vi "free tls config.vi"(8 "error in":errorcluster, 11 "config":u64) -> (0 "error out":errorcluster)   [LabVIEW 2016, in "lv tls dll.lvlib"]
uses:
  lv tls dll.lvlib
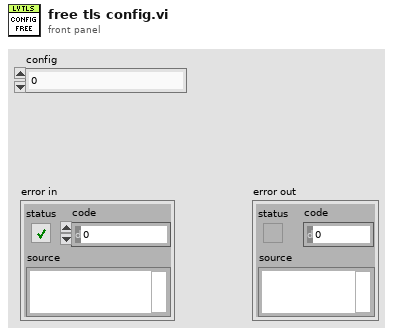
[diagram p1: front panel]
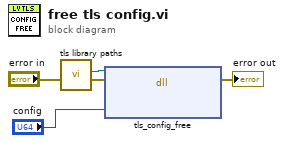
[diagram p0: block diagram]
diagram:
  n1 = call "tls library paths.vi"() -> ("libtls"=w4:path)  [unwired: 8 in, 3 out]
  n2 = dll-call lib="C:/Users/IEUser/Desktop/tlssimple/libtls-15.dll" fn="tls_config_free"(path in=w4, error in="error in", "config"="config") -> (error out=→"error out":errorcluster)  [unwired: 3 in, 1 out]
